vi "WriteDataMethod.vi"(8 "Error In":errorcluster, 10 "Data Method":refnum<class "IDataMethod.lvclass">, 11 "object in":refnum<class "DataType.lvclass">) -> (0 "Error Out":errorcluster, 3 "object out":refnum<class "DataType.lvclass">)   [LabVIEW 2024, in "DataType.lvclass"]
uses:
  <resource>/Framework/Providers/Open_GDS/ClassProviders/Provider_LvNativeClass/Templates/NativeBaseTemplate/NativeBaseTemplate.lvclass/NativeBaseTemplate.ctl
  DataType.lvclass
  DataType.lvclass/DataType.ctl
  IDataMethod_interface/IDataMethod.lvclass
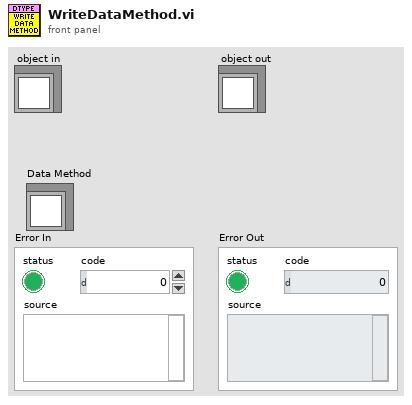
[diagram p1: front panel]
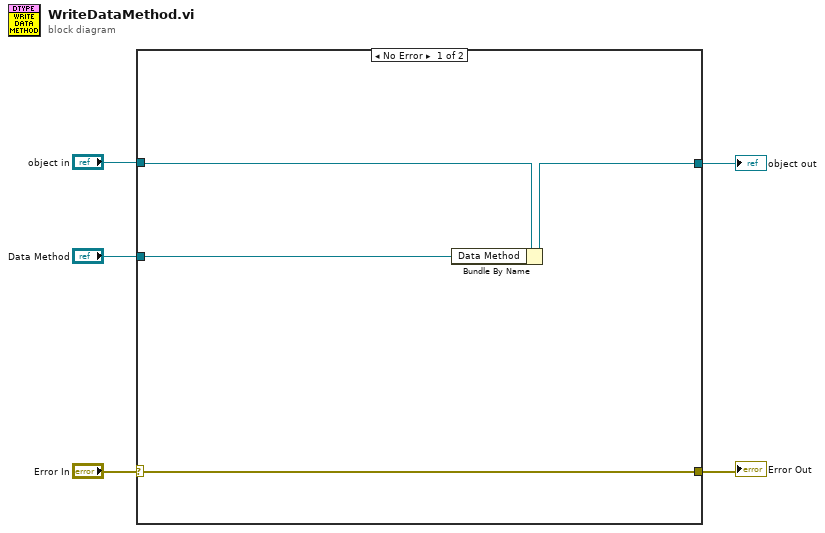
[diagram p0: block diagram]
diagram:
  n1 = case shown="No Error" "Error In" {
    selector: "Error In" -> [w8 w11]
    tunnel: [w8 w11] -> w4
    tunnel: [w6 w10] -> w2
    tunnel: "object in" -> [w7 w10]
    tunnel: "Data Method" -> [w9 _]
    frame No Error {
      n2 = Bundle By Name(cluster=w7, "Data Method"=w9) -> (w6:refnum<class "DataType.lvclass">)
    }
    frame Error {
    }
  }
  "Error Out" <- w4
  "object out" <- w2
